vi "fecth_cu_keyvalue.vi"(9 "cuname":string, 11 "handleConnection":u32) -> (0 "data out":string[](array[string]), 1 "timestemp":string, 2 "CU name":string, 3 "tot of buf word":i32, 4 "String data out":string, 5 "values out":string)   [LabVIEW 2014]
uses:
  common/crest/LabVIEW/LV14/libcommon-crest.lvlib
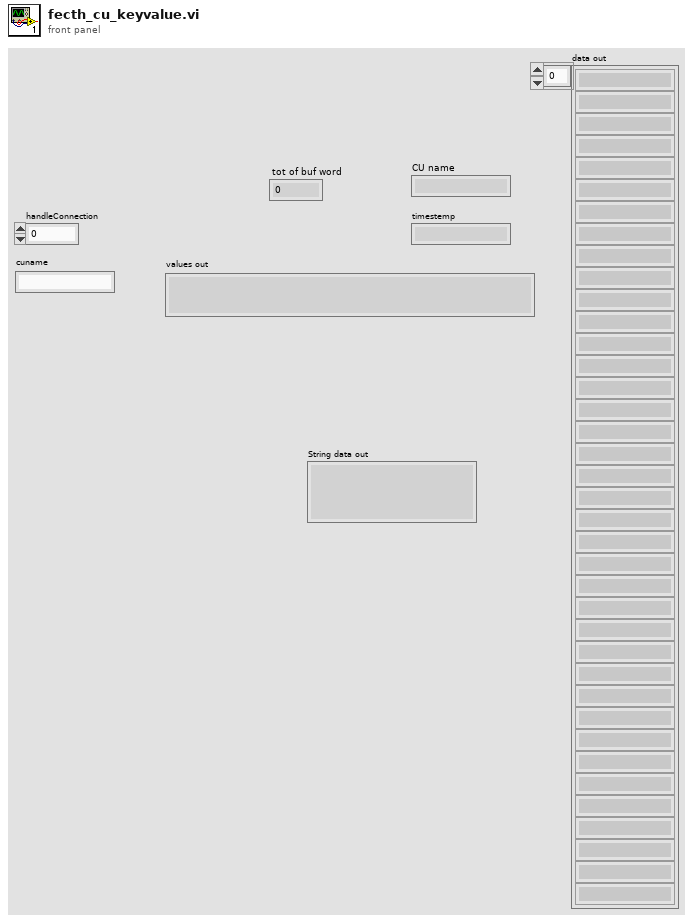
[diagram p1: front panel]
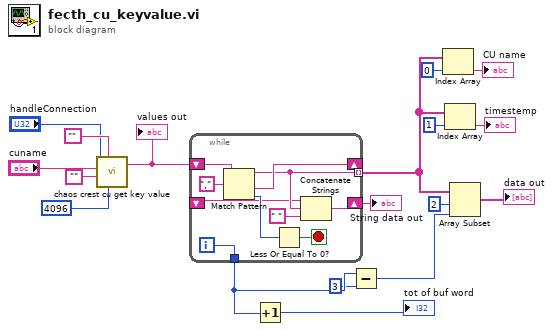
[diagram p0: block diagram]
diagram:
  n1 = call "chaos crest cu get key value.vi"("maxsize"=4096, "values"="", "keys"="", "cuname"="cuname", "handleConnection"="handleConnection") -> ("values out"=w15:string)  [unwired: 3 in, 3 out]
  "values out" <- w15
  n2 = while {
    shift-right: [w23] -> _
    shift-left: w15 -> [w27]
    tunnel: [w21] -> w9 mode=indexing
    tunnel: [w24] -> w7
    shift-right: [w20] -> w1
    shift-left: _ -> [w19]
    i -> [w24]
    stop <- w26 stop-if-true
    n3 = Match Pattern(string=w27, regular expression=",") -> (before substring=w21:string, after substring=w23:string, offset past match=w25:i32)  [unwired: 1 in, 1 out]
    n4 = Less Or Equal To 0?(x=w25) -> (x <= 0?=w26:bool)
    n5 = Concatenate Strings(w19, w21, " " ("element")) -> (w20:string)
  }
  "String data out" <- w1
  n6 = Increment(x=w7) -> (x+1=→"tot of buf word":i32)
  n7 = Subtract(x=w7, y=3) -> (x-y=w5:i32)
  n8 = Index Array(array=w9, index=0) -> (element=→"CU name":string)
  n9 = Index Array(array=w9, index=1) -> (element=→"timestemp":string)
  n10 = Array Subset(array=w9, index=2, length=w5) -> (→"data out":string[])
